vi "Sound.vi"(11 "Input":string) -> ()   [LabVIEW 2023]
panel:
  out "Waveform Graph":waveform(dbl)(graph)
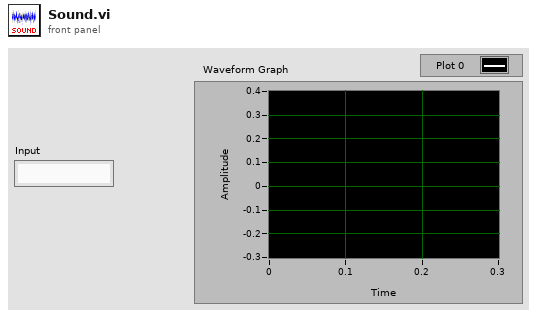
[diagram p1: front panel]
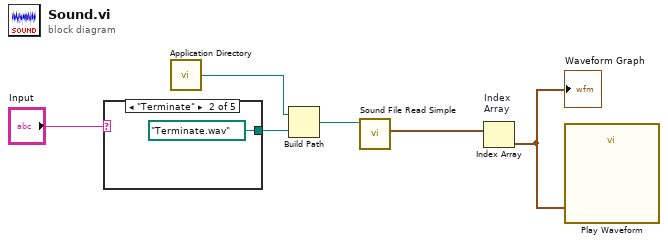
[diagram p0: block diagram]
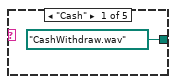
[diagram p2: hidden frame]
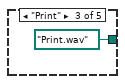
[diagram p3: hidden frame]
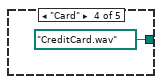
[diagram p4: hidden frame]
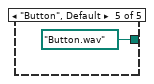
[diagram p5: hidden frame]
diagram:
  n1 = case shown="\"Terminate\"" "Input" {
    tunnel: [path "CashWithdraw.wav" ("name or relative path") path "Terminate.wav" ("name or relative path") path "Print.wav" ("name or relative path") path "CreditCard.wav" ("name or relative path") path "Button.wav" ("name or relative path")] -> w1
    frame "Cash" {
    }
    frame "Terminate" {
    }
    frame "Print" {
    }
    frame "Card" {
    }
    frame "Button", Default {
    }
  }
  n2 = call <vilib>:"Application Directory.vi"() -> ("Application Directory"=w6:path)
  n3 = Build Path(base path=w6, name or relative path=w1) -> (appended path=w5:path)
  n4 = call <vilib>:"Sound File Read Simple.vi"("path"=w5) -> ("data"=w4:waveform(dbl)[])  [unwired: 7 in, 3 out]
  n5 = Index Array "Index \nArray"(array=w4) -> (element=w3:waveform(dbl))  [unwired: 1 in]
  "Waveform Graph" <- w3
  n6 = call "Play Waveform"("Data"=w3) -> ()  [unwired: 18 in, 1 out]
